vi "CD Init_Prepare Async Data_RTs Status.vi"(8 "error in (no error)":errorcluster, 10 "Card Parameters (in)":T1, 11 "Channels In":T7[](array[typedef]) {"RTs"."Mode Codes"."Words Item Refs" format="%.0x"; "RTs"."Mode Codes"."Timestamp Channel Data Reference" format="%.0x"; "RTs"."subAddresses"."Words Item Refs" format="%.0x"; "RTs"."subAddresses"."Timestamp Channel Data Reference" format="%.0x"; "RTs"."Status Channel Data Reference" format="%.0x"; "RTs"."Command Channels Refs" format="%.0x"; "BC"."Acyclic Frames Trigger Channels Refs" format="%.0x"; "BC"."Command Channels Refs" format="%.0x"; "BC"."messages"."Timestamp Channel Data Reference" format="%.0x"; "BC"."messages"."Status Channel Data Refs" format="%.0x"; "BC"."messages"."Words Item Refs" format="%.0x"; "BC"."messages"."Words Block Data Refs"."Data Reference" format="%.0x"}) -> (0 "error out":errorcluster, 2 "Raw Values (RTs Status)":T3, 3 "Map (RTs Status)":T5[](array[typedef]))   [LabVIEW 2017, in "Ballard MIL-1553 Engine.lvlib"]
doc: "This VI creates a static association between NI-VS FIFO Channel Index and Physical Channel, Label Index, Parameter Index for Parameter Channel of a Tx Scheduled Label."
uses:
  Ballard MIL-1553 Engine.lvlib
  Shared/Controls and Global/RT Channel.ctl
  Shared/Controls and Global/RT BC.ctl
  <vilib>/NI Veristand/Custom Device API/Custom Device Item Ref.ctl
  Shared/Controls and Global/RT Message.ctl
  Shared/Controls and Global/RT messageType.ctl
  Shared/Controls and Global/RT CWD1.ctl
  Shared/Controls and Global/RT CWD2.ctl
  <vilib>/NI Veristand/Custom Device API/Data Reference.ctl
  <vilib>/NI Veristand/Custom Device API/Block Data Reference.ctl
  Shared/Controls and Global/RT Remote Terminal.ctl
  Shared/Controls and Global/RT Remote Terminal_rtMode.ctl
  Shared/Controls and Global/RT Remote Terminal_RT subAddress.ctl
  Shared/Controls and Global/RT Remote Terminal_RT direction.ctl
  Shared/Controls and Global/RT Remote Terminal_RT Mode Code.ctl
  Controls/RT Async_Map RTs Status.ctl
  Controls/RT Async_Map_Type.ctl
  Controls/RT Async_Raw Values.ctl
  Controls/RT Async_Raw Values to Messages Index_Association.ctl
  Controls/Card Parameters.ctl
  Shared/Controls and Global/Initialization Method.ctl
  Controls/RT Async_Raw Values_Association.ctl
  <vilib>/NI VeriStand/Custom Device API/Custom Device API.lvlib
  <instrlib>/BTI1553Lib/BTI1553LV.lvlib
  Shared/Ballard 1553 Shared.lvlib
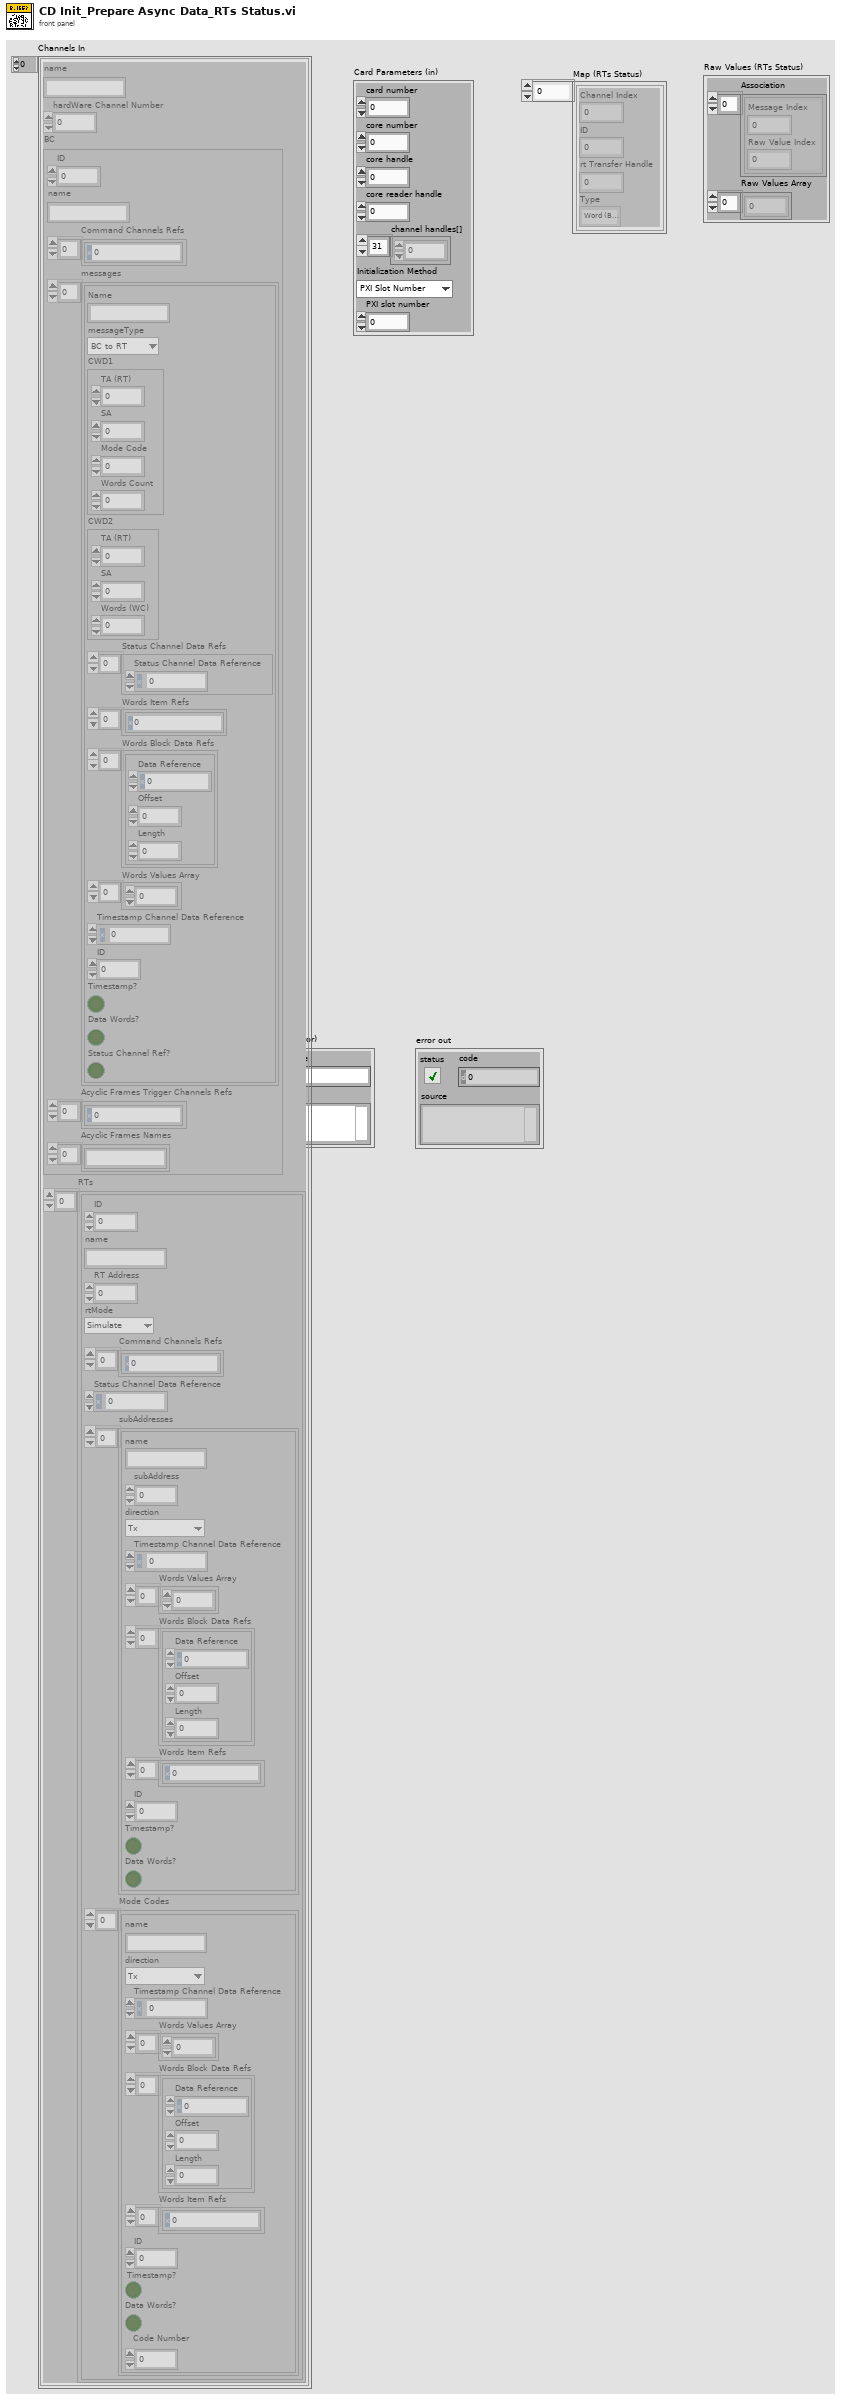
[diagram p1: front panel]
types:
  T1 = typedef "Ballard MIL-1553 Engine.lvlib/Card Parameters.ctl" = cluster{"card number":i32, "core number":i32, "core handle":u64, "core reader handle":u64, "channel handles[]":u64[], "Initialization Method":T2, "PXI slot number":i32}
  T2 = typedef "Ballard 1553 Shared.lvlib/Initialization Method.ctl" = enum16{"PXI Slot Number", "Card Number"}
  T3 = typedef "Ballard MIL-1553 Engine.lvlib/RT Async_Raw Values.ctl" = cluster{"Association":T4[], "Raw Values Array":u16[]}
  T4 = typedef "Ballard MIL-1553 Engine.lvlib/RT Async_Raw Values to Messages Index_Association.ctl" = cluster{"Message Index":i32, "Raw Value Index":i32}
  T5 = typedef "Ballard MIL-1553 Engine.lvlib/RT Async_Map RTs Status.ctl" = cluster{"Channel Index":i32, "ID":i32, "rt Transfer Handle":u64, "Type":T6}
  T6 = typedef "Ballard MIL-1553 Engine.lvlib/RT Async_Map_Type.ctl" = enum16{"Word (BC to RT)", "Word (MC (Rx))", "Acyclic Message Trigger", "Word (RT to ..)", "Word (RT to RT)", "Word (MC (Tx))", "RT Status", "BC Commands", "RT Commands"}
  T7 = typedef "Ballard 1553 Shared.lvlib/RT Channel.ctl" = cluster{"name":string, "hardWare Channel Number":u16, "BC":T8, "RTs":T16[]}
  T8 = typedef "Ballard 1553 Shared.lvlib/RT BC.ctl" = cluster{"ID":i32, "name":string, "Command Channels Refs":T9[], "messages":T10[], "Acyclic Frames Trigger Channels Refs":T9[], "Acyclic Frames Names":string[]}
  T9 = typedef "Custom Device API.lvlib/Custom Device Item Ref.ctl" = u64
  T10 = typedef "Ballard 1553 Shared.lvlib/RT Message.ctl" = cluster{"Name":string, "messageType":T11, "CWD1":T12, "CWD2":T13, "Status Channel Data Refs":T14[], "Words Item Refs":T9[], "Words Block Data Refs":T15[], "Words Values Array":u16[], "Timestamp Channel Data Reference":T14, "ID":i32, "Timestamp?":bool, "Data Words?":bool, "Status Channel Ref?":bool}
  T11 = typedef "Ballard 1553 Shared.lvlib/RT messageType.ctl" = enum16{"BC to RT", "RT to BC", "RT to RT", "MC (Rx)", "MC (Tx)"}
  T12 = typedef "Ballard 1553 Shared.lvlib/RT CWD1.ctl" = cluster{"TA (RT)":i8, "SA":i8, "Mode Code":i8, "Words Count":i8}
  T13 = typedef "Ballard 1553 Shared.lvlib/RT CWD2.ctl" = cluster{"TA (RT)":i8, "SA":i8, "Words (WC)":i8}
  T14 = typedef "Custom Device API.lvlib/Data Reference.ctl" = i32
  T15 = typedef "Custom Device API.lvlib/Block Data Reference.ctl" = cluster{"Data Reference":T14, "Offset":u64, "Length":u64}
  T16 = typedef "Ballard 1553 Shared.lvlib/RT Remote Terminal.ctl" = cluster{"ID":i32, "name":string, "RT Address":i32, "rtMode":T17, "Command Channels Refs":T9[], "Status Channel Data Reference":T14, "subAddresses":T18[], "Mode Codes":T20[]}
  T17 = typedef "Ballard 1553 Shared.lvlib/RT Remote Terminal_rtMode.ctl" = enum16{"Simulate", "Monitor", "Disable"}
  T18 = typedef "Ballard 1553 Shared.lvlib/RT Remote Terminal_RT subAddress.ctl" = cluster{"name":string, "subAddress":i8, "direction":T19, "Timestamp Channel Data Reference":T14, "Words Values Array":u16[], "Words Block Data Refs":T15[], "Words Item Refs":T9[], "ID":i32, "Timestamp?":bool, "Data Words?":bool}
  T19 = typedef "Ballard 1553 Shared.lvlib/RT Remote Terminal_RT direction.ctl" = enum16{"Tx", "Rx"}
  T20 = typedef "Ballard 1553 Shared.lvlib/RT Remote Terminal_RT Mode Code.ctl" = cluster{"name":string, "direction":T19, "Timestamp Channel Data Reference":T14, "Words Values Array":u16[], "Words Block Data Refs":T15[], "Words Item Refs":T9[], "ID":i32, "Timestamp?":bool, "Data Words?":bool, "Code Number":i32}
  T21 = typedef "Ballard MIL-1553 Engine.lvlib/RT Async_Raw Values_Association.ctl" = cluster{"Channel Data Reference":T14, "Raw Value Index":i32}
  T22 = typedef "Custom Device API.lvlib/Custom Device Channel.ctl" = cluster{"Type":T23, "Units":string, "Default Value":dbl, "Faultable":bool, "Scalable":bool}
  T23 = typedef "Custom Device API.lvlib/Custom Device Channel Type.ctl" = enum16{"Input", "Output"}
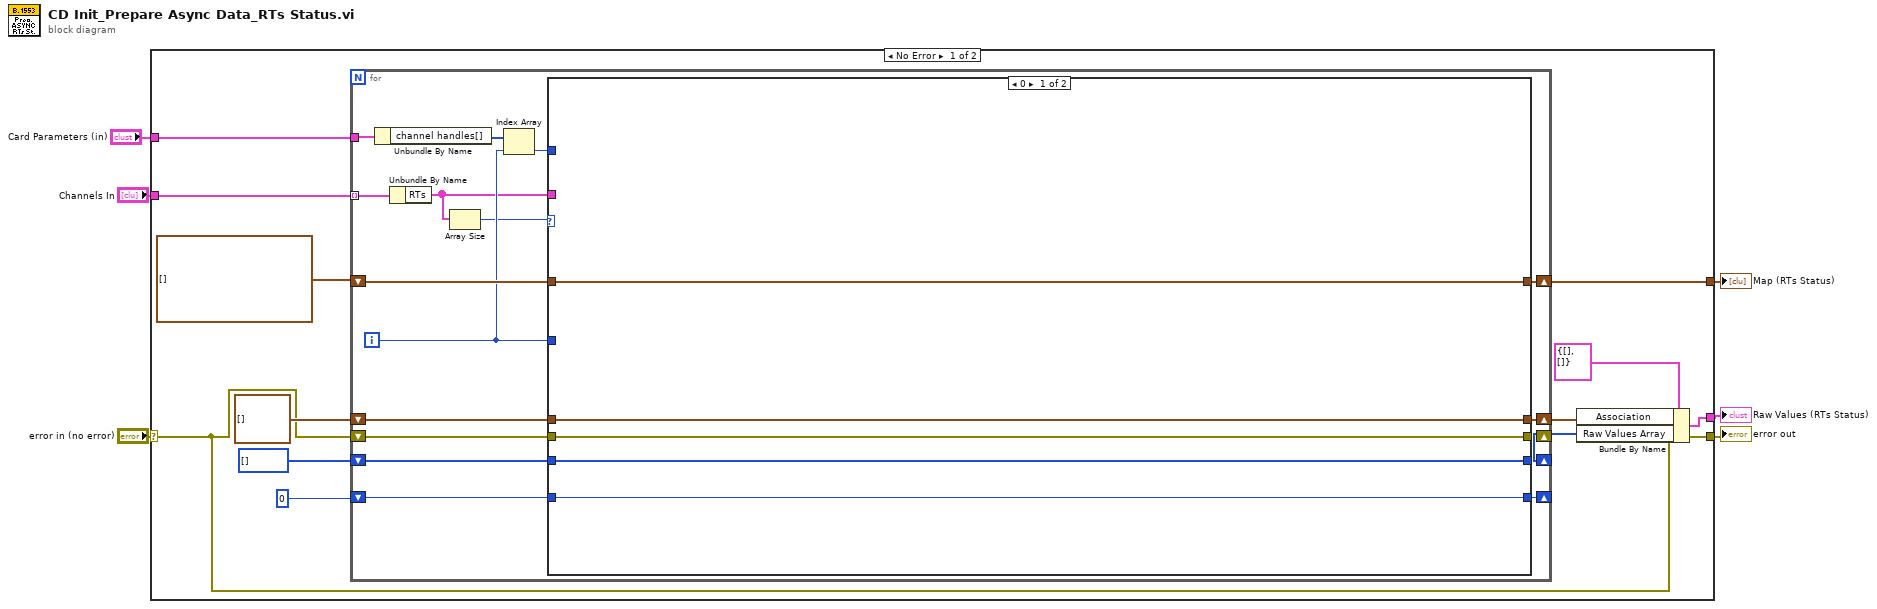
[diagram p0: block diagram]
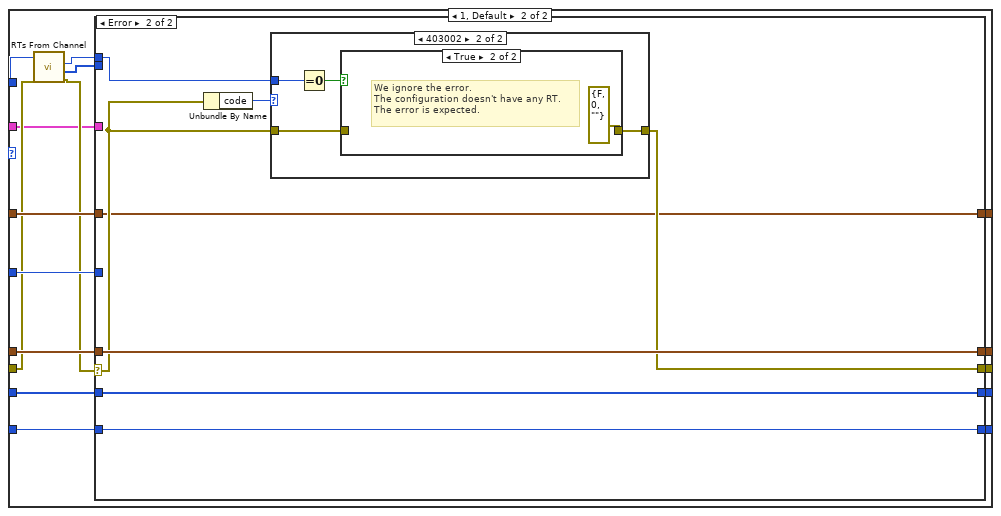
[diagram p2: hidden frame]
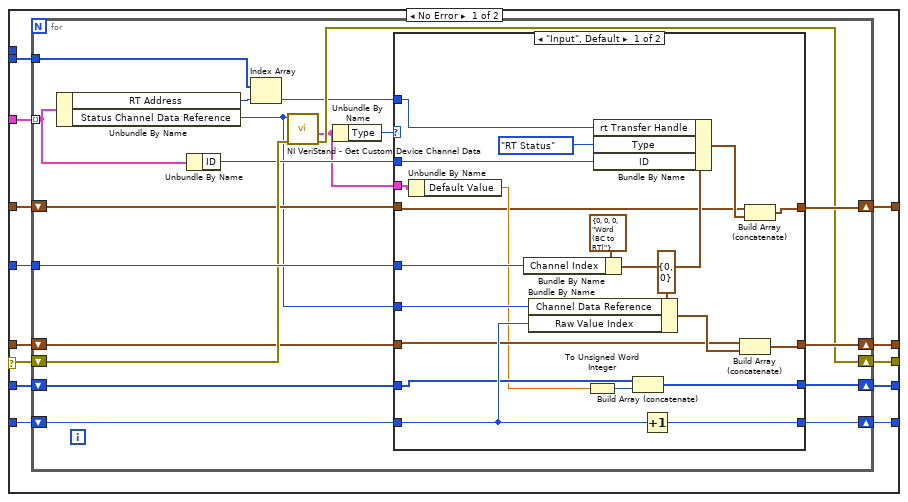
[diagram p3: hidden frame]
diagram:
  n1 = case shown="No Error" "error in (no error)" {
    selector: "error in (no error)" -> [w7 w129]
    tunnel: [w7 w129] -> w5
    tunnel: "Channels In" -> [w18 _]
    tunnel: [w16 _] -> w3
    tunnel: [w12 _] -> w2
    tunnel: "Card Parameters (in)" -> [w8 _]
    frame No Error {
      n2 = for {
        tunnel: w18 -> [w35] mode=indexing
        shift-right: [w33] -> w16
        shift-left: T5[] [] -> [w34]
        shift-right: [w31] -> w13
        shift-left: T21[] [] -> [w32]
        shift-right: [w27] -> w10
        shift-left: u16[] [] -> [w30]
        shift-right: [w28] -> _
        shift-left: 0 -> [w29]
        tunnel: w8 -> [w26]
        shift-right: [w23] -> _
        shift-left: w7 -> [w21]
        i -> [w24]
        n3 = Unbundle By Name(w26) -> ("channel handles[]"=w25:u64[])
        n4 = Unbundle By Name(w35) -> ("RTs"=w20:T16[])
        n5 = Array Size(array=w20) -> (size(s)=w19:i32)
        n6 = Index Array(array=w25, index=w24) -> (element=w22:u64)
        n7 = case shown="0" w19 {
          tunnel: w34 -> [w40 w56]
          tunnel: [w40 w55] -> w33
          tunnel: w32 -> [w39 w54]
          tunnel: [w39 w53] -> w31
          tunnel: w30 -> [w37 w52]
          tunnel: w29 -> [w36 w51]
          tunnel: [w36 w50] -> w28
          tunnel: [w37 w49] -> w27
          tunnel: w24 -> [_ w48]
          tunnel: [w38 w47] -> w23
          tunnel: w22 -> [_ w46]
          tunnel: w21 -> [w38 w45]
          tunnel: w20 -> [_ w41]
          frame 0 {
          }
          frame 1, Default {
            n8 = call <instrlib>:"RTs From Channel.vi"("error in (no error)"=w45, "channel handle in"=w46) -> ("error out"=w43:errorcluster, "remote terminal handles out"=w44:u64[], "remote terminal count out"=w42:i32)  [unwired: 6 in, 1 out]
            n9 = case shown="Error" w43 {
              selector: w43 -> [w57 w117]
              tunnel: w41 -> [w69 _]
              tunnel: w56 -> [w68 w114]
              tunnel: [w67 w114] -> w55
              tunnel: w54 -> [w66 w120]
              tunnel: [w65 w120] -> w53
              tunnel: w52 -> [w64 w119]
              tunnel: w51 -> [w63 w118]
              tunnel: [w62 w118] -> w50
              tunnel: [w61 w119] -> w49
              tunnel: w48 -> [w60 _]
              tunnel: [w59 w115] -> w47
              tunnel: w44 -> [w58 _]
              tunnel: w42 -> [_ w116]
              frame No Error {
                n10 = for {
                  tunnel: w69 -> [w76] mode=indexing
                  shift-right: [w87] -> w67
                  shift-left: w68 -> [w78]
                  tunnel: w60 -> [w88]
                  shift-right: [w86] -> w65
                  shift-left: w66 -> [w77]
                  shift-right: [w85] -> w61
                  shift-left: w64 -> [w82]
                  shift-right: [w84] -> w62
                  shift-left: w63 -> [w83]
                  tunnel: w58 -> [w71]
                  shift-right: [w79] -> w59
                  shift-left: w57 -> [w81]
                  n11 = Unbundle By Name(w76) -> ("RT Address"=w72:i32, "Status Channel Data Reference"=w74:T14)
                  n12 = Unbundle By Name(w76) -> ("ID"=w75:i32)
                  n13 = Index Array(array=w71, index=w72) -> (element=w70:u64)
                  n14 = call <vilib>:"NI VeriStand - Get Custom Device Channel Data.vi"("error in (no error)"=w81, "Channel Ref in"=w74) -> ("error out"=w79:errorcluster, "Channel"=w73:T22)  [unwired: 4 in, 4 out]
                  n15 = Unbundle By Name(w73) -> ("Type"=w80:T23)
                  n16 = case shown="\"Input\", Default" w80 {
                    tunnel: w88 -> [w109 _]
                    tunnel: [w108 w113] -> w87
                    tunnel: [w107 w112] -> w86
                    tunnel: [w106 w111] -> w85
                    tunnel: [w105 w110] -> w84
                    tunnel: w83 -> [w104 w110]
                    tunnel: w82 -> [w103 w111]
                    tunnel: w78 -> [w90 w113]
                    tunnel: w77 -> [w93 w112]
                    tunnel: w75 -> [w96 _]
                    tunnel: w74 -> [w95 _]
                    tunnel: w73 -> [w94 _]
                    tunnel: w70 -> [w89 _]
                    frame "Input", Default {
                      n17 = Unbundle By Name(w94) -> ("Default Value"=w91:dbl)
                      n18 = Bundle By Name(cluster=T5 {"Channel Index"=0, "ID"=0, "rt Transfer Handle"=0, "Type"=enum."Word (BC to RT)"} ("Association"), "Channel Index"=w109) -> (w102:T5)
                      n19 = Bundle By Name(cluster=T21 {"Channel Data Reference"=0, "Raw Value Index"=0}, "Channel Data Reference"=w95, "Raw Value Index"=w104) -> (w99:T21)
                      n20 = To Unsigned Word Integer(number=w91) -> (unsigned 16bit integer=w92:u16)
                      n21 = Bundle By Name(cluster=w102, "rt Transfer Handle"=w89, "Type"=RT_Async_Map_Type."RT Status", "ID"=w96) -> (w98:T5)
                      n22 = Build Array (concatenate)(w103, w92) -> (w106:u16[])
                      n23 = Increment(x=w104) -> (x+1=w105:i32)
                      n24 = Build Array (concatenate)(w93, w99) -> (w107:T21[])
                      n25 = Build Array (concatenate)(w90, w98) -> (w108:T5[])
                    }
                    frame "Output" {
                    }
                  }
                }
              }
              frame Error {
                n26 = Unbundle By Name(w117) -> ("code"=w121:i32)
                n27 = case shown="403002" w121 {
                  tunnel: w117 -> [w122 w124]
                  tunnel: w116 -> [_ w126]
                  tunnel: [w122 w123] -> w115
                  frame 0, Default {
                  }
                  frame 403002 {
                    n28 = Equal To 0?(x=w126) -> (x = 0?=w125:bool)
                    n29 = case shown="True" w125 {
                      tunnel: w124 -> [w127 _]
                      tunnel: [w127 errorcluster {"status"=FALSE, "code"=0, "source"=""} ("error IO")] -> w123
                      frame False {
                      }
                      frame True {
                        # "We ignore the error.\nThe configuration doesn't have any RT.\nThe error is expected."
                      }
                    }
                  }
                }
              }
            }
          }
        }
      }
      n30 = Bundle By Name(cluster=T3 {"Association"=[], "Raw Values Array"=[]} ("Raw Values"), "Association"=w13, "Raw Values Array"=w10) -> (w12:T3)
    }
    frame Error {
    }
  }
  "error out" <- w5
  "Map (RTs Status)" <- w3
  "Raw Values (RTs Status)" <- w2
